vi "Set_Height.vi"(8 "error in (no error)":errorcluster caption="错误输入（无错误）", 10 "Height":dbl, 11 "Size输入":refnum<class "Size.lvclass">) -> (0 "error out":errorcluster caption="错误输出", 3 "Size输出":refnum<class "Size.lvclass">)   [LabVIEW 2011, in "Size.lvclass"]
uses:
  Size.lvclass
  Size.lvclass/Size.ctl
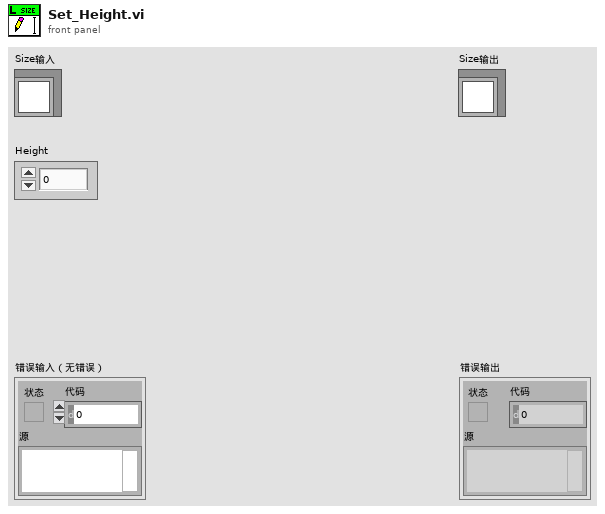
[diagram p1: front panel]
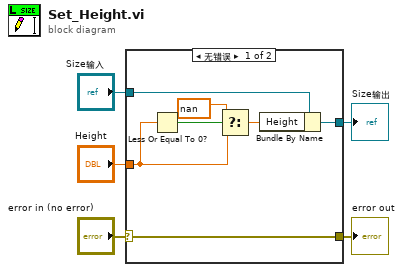
[diagram p0: block diagram]
diagram:
  n1 = case shown="无错误" "error in (no error)" {
    selector: "error in (no error)" -> [w12 w13]
    tunnel: [w12 w13] -> w4
    tunnel: [w10 w14] -> w2
    tunnel: "Size输入" -> [w11 w14]
    tunnel: "Height" -> [w7 _]
    frame No Error {
      n2 = Less Or Equal To 0?(x=w7) -> (x <= 0?=w9:bool)
      n3 = Select(t=nan, s=w9, f=w7) -> (s? t:f=w6:dbl)
      n4 = Bundle By Name(cluster=w11, "Height"=w6) -> (w10:refnum<class "Size.lvclass">)
    }
    frame Error {
    }
  }
  "error out" <- w4
  "Size输出" <- w2
